vi "move_multi.vi"() -> ()   [LabVIEW 2023]
panel:
  out "torque":dbl[](array[numeric])
  out "position":dbl[](array[numeric])
  out "Start Error":errorcluster
  out "Main Error":errorcluster
  in  "?":bool
  in  "Positon Inputs":dbl[](array[numeric])
  in  "Number of Motors":i64
  # "Multi Motor Move"
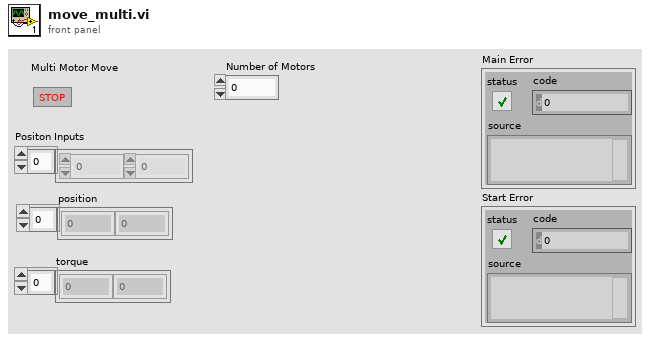
[diagram p1: front panel]
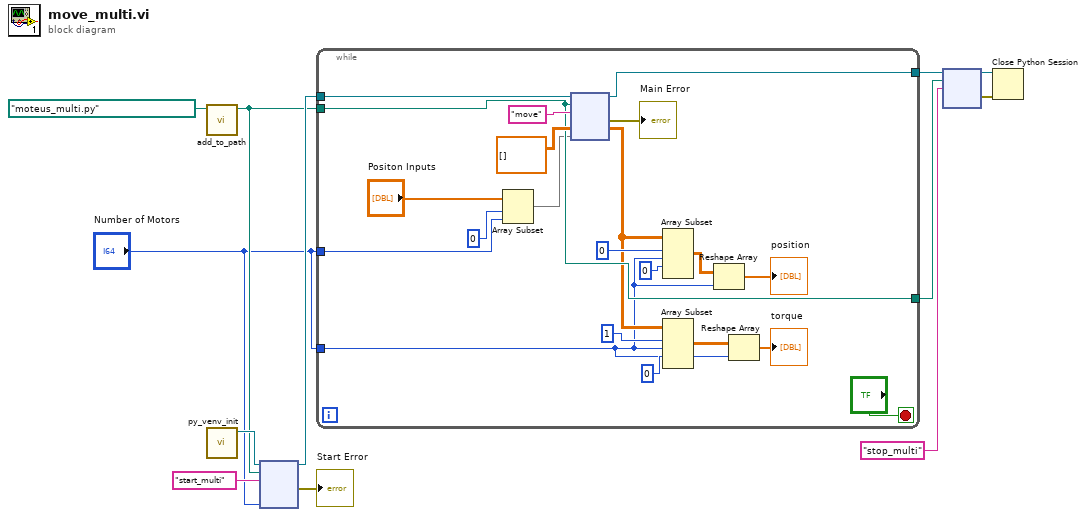
[diagram p0: block diagram]
diagram:
  n1 = call "add_to_path.vi"("Path"=path "moteus_multi.py") -> ("appended path"=w8:path)  [unwired: 10 in]
  n2 = call "py_venv_init.vi"() -> ("Refnum out"=w11:refnum<k35>)  [unwired: 11 in]
  n3 = node(w11, w8, "start_multi", "Number of Motors") -> (w9:refnum<k35>, →"Start Error":errorcluster)  [unwired: 4 in, 2 out]
  n4 = while {
    tunnel: w9 -> [w33]
    tunnel: w8 -> [w28]
    tunnel: [w29] -> w7
    tunnel: [w28] -> w6
    tunnel: "Number of Motors" -> [w13]
    tunnel: "Number of Motors" -> [w17]
    stop <- "?" stop-if-true
    n5 = Array Subset(array="Positon Inputs", index=0, length=w17) -> (w16:dbl[])
    n6 = node(w33, w28, "move", dbl[][] [], w16) -> (w29:refnum<k35>, →"Main Error":errorcluster, w24:dbl[][])  [unwired: 2 in, 2 out]
    n7 = Array Subset(array=w24, index (row)=0, length (row)=w13, index (col)=0) -> (w21:dbl[][])  [unwired: 1 in]
    n8 = Array Subset(array=w24, index (row)=1, length (row)=w13, index (col)=0) -> (w18:dbl[][])  [unwired: 1 in]
    n9 = Reshape Array(w21, w13) -> (→"position":dbl[])
    n10 = Reshape Array(w18, w13) -> (→"torque":dbl[])
  }
  n11 = node(w7, w6, "stop_multi") -> (w3:refnum<k35>, w2:errorcluster)  [unwired: 3 in, 2 out]
  n12 = Close Python Session(session in=w3, error in=w2) -> ()  [unwired: 1 out]
